vi "Set Target Project.vi"(8 "error in (no error)":errorcluster, 9 "Target Project":string(combo), 10 "Projects":T1, 11 "ComboBox Ref":refnum<vi>) -> (0 "error out":errorcluster)   [LabVIEW 2015, in "Configuration Tool.lvlib"]
uses:
  Configuration Tool.lvlib
  Global Settings.vi
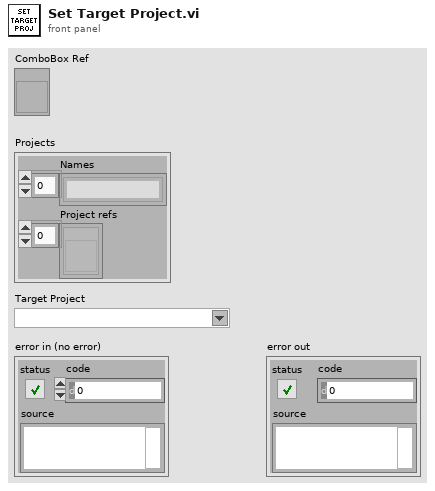
[diagram p1: front panel]
types:
  T1 = cluster{"Names":string[], "Project refs":refnum<vi>[]}
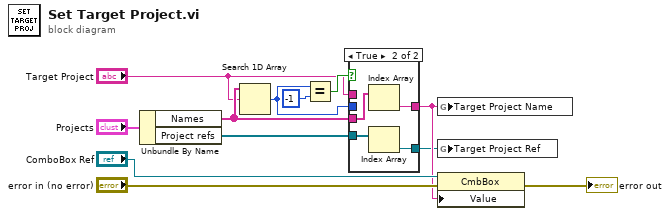
[diagram p0: block diagram]
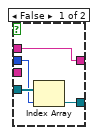
[diagram p2: hidden frame]
diagram:
  n1 = Unbundle By Name("Projects") -> ("Names"=w8:string[], "Project refs"=w2:refnum<vi>[])
  n2 = Search 1D Array(1D array=w8, element="Target Project") -> (index of element=w3:i32)  [unwired: 1 in]
  n3 = Equal?(x=w3, y=-1) -> (x = y?=w6:bool)
  n4 = case shown="True" w6 {
    tunnel: [w16 w19] -> w5
    tunnel: "Target Project" -> [w16 _]
    tunnel: [w13 w17] -> w1
    tunnel: w8 -> [_ w20]
    tunnel: w2 -> [w15 w18]
    tunnel: w3 -> [w14 _]
    frame False {
      n5 = Index Array(array=w15, index=w14) -> (element=w13:refnum<vi>)
    }
    frame True {
      n6 = Index Array(array=w20) -> (element=w19:string)  [unwired: 1 in]
      n7 = Index Array(array=w18) -> (element=w17:refnum<vi>)  [unwired: 1 in]
    }
  }
  n8 = global write "Global Settings.vi" "Target Project Name"(w5) -> ()
  n9 = global write "Global Settings.vi" "Target Project Ref"(w1) -> ()
  n10 = property class="CmbBox"(reference="ComboBox Ref", error in="error in (no error)", "Value"=w5) -> (error out=→"error out":errorcluster)  [unwired: 1 out]
